vi "搜索所有匹配元素(2D---1D I16).vi"(8 "error in (no error)":errorcluster caption="错误输入（无错误）", 9 "开始索引（0）":i32, 10 "元素":i16, 11 "数组":i16[][](array[numeric])) -> (0 "error out":errorcluster caption="错误输出", 1 "匹配数量":i32, 3 "匹配元素索引":cluster{"行":i32, "列":i32}[](array[cluster]))   [LabVIEW 2011]
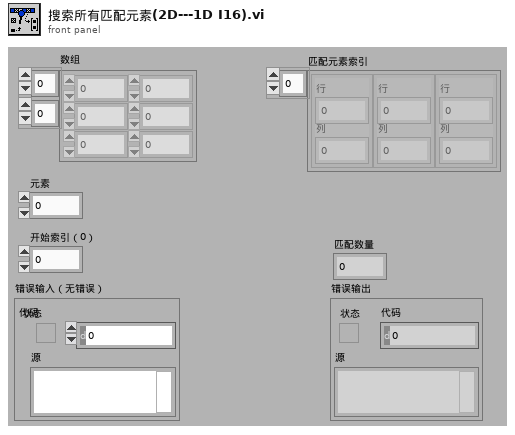
[diagram p1: front panel]
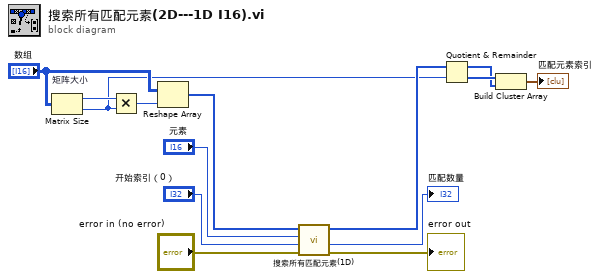
[diagram p0: block diagram]
diagram:
  n1 = Matrix Size "矩阵大小"(0:"数组") -> (1:w13:i32, 2:w4:i32)
  n2 = Multiply(x=w13, y=w4) -> (x*y=w12:i32)
  n3 = Reshape Array("数组", w12) -> (w11:i16[])
  n4 = call-poly "搜索所有匹配元素(1D).vi"("error in (no error)"="error in (no error)", "开始索引（0）"="开始索引（0）", "元素"="元素", "数组"=w11) -> ("error out"=→"error out":errorcluster, "匹配数量"=→"匹配数量":i32, "匹配元素索引"=w5:i32[])  [unwired: 5 in]
  n5 = Quotient & Remainder(x=w5, y=w4) -> (x-y*floor(x/y)=w2:i32[], floor(x/y)=w3:i32[])
  n6 = Build Cluster Array(w3, w2) -> (→"匹配元素索引":cluster{i32, i32}[])
